vi "LS372_only_readout_Monitor.vi"() -> ()   [LabVIEW 2019]
uses:
  Utility/LS372/LS372_read_only-Cluster.ctl
  Global/Global Variables/Data_Display_global.vi
  Instrument_Setup.vi
  Equipment/Lake Shore 372/Lake Shore 372.lvlib
panel:
  in  "stop":bool
  out "LS372_only_read-Cluster":T1
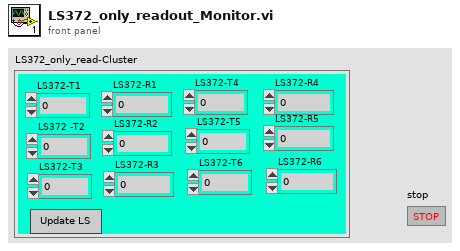
[diagram p1: front panel]
types:
  T1 = typedef "LS372_read_only-Cluster.ctl" = cluster{"LS372-T1":dbl, "LS372 -T2":dbl, "LS372-T4":dbl, "LS372-T5":dbl, "LS372-T6":dbl, "LS372-R1 ":dbl, "LS372-R2":dbl, "LS372-R3 ":dbl, "LS372-R4 \n\n\n\n":dbl, "LS372-R5":dbl, "LS372-R6 ":dbl, "LS372-T3":dbl, "Update Lakeshores":bool}
  T2 = typedef "LS372_read_only-Control.ctl" = cluster{"Update Lakeshores":bool}
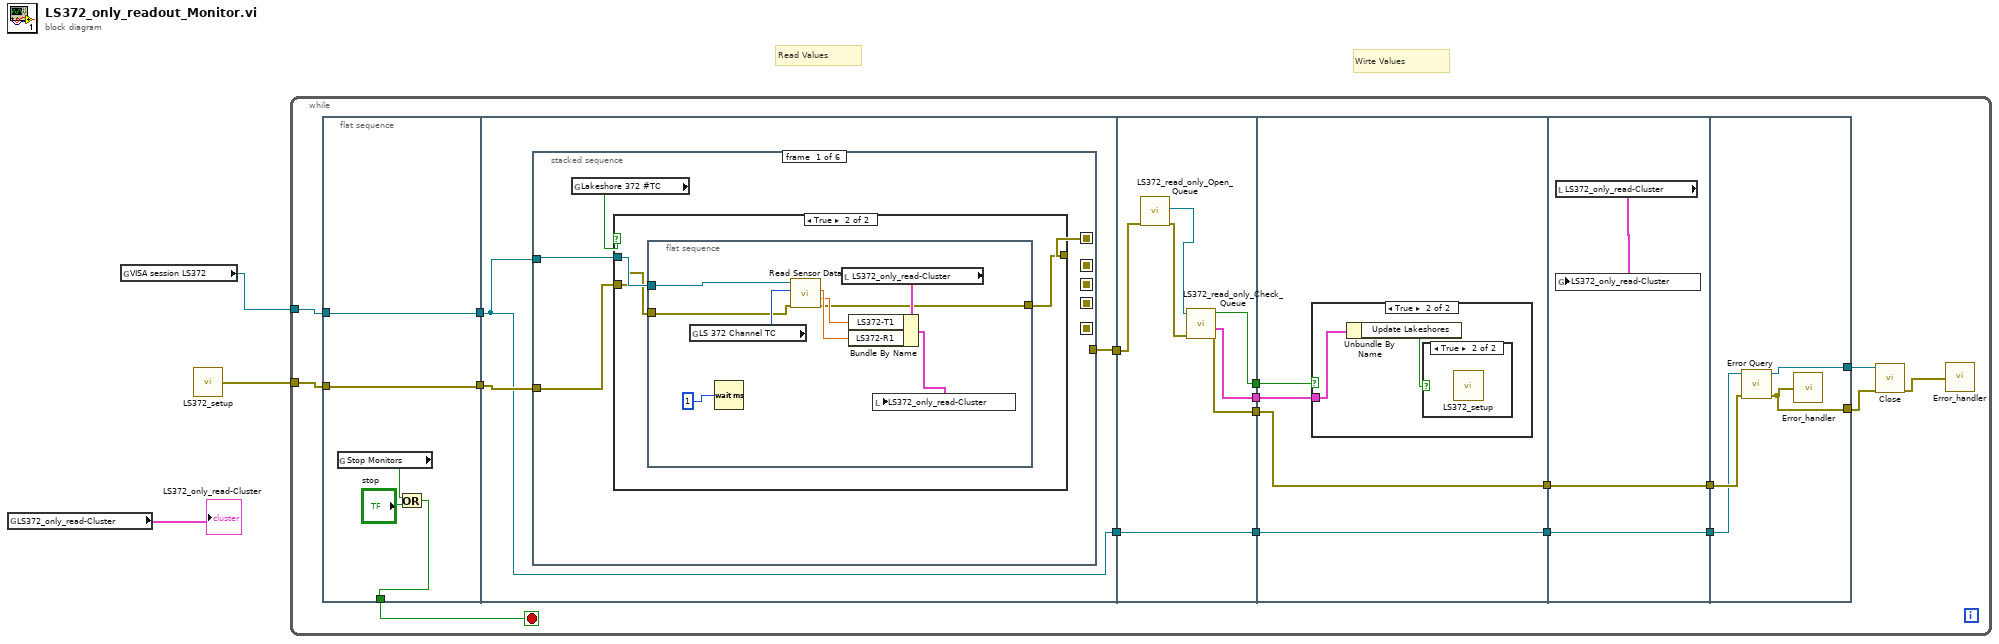
[diagram p0: block diagram]
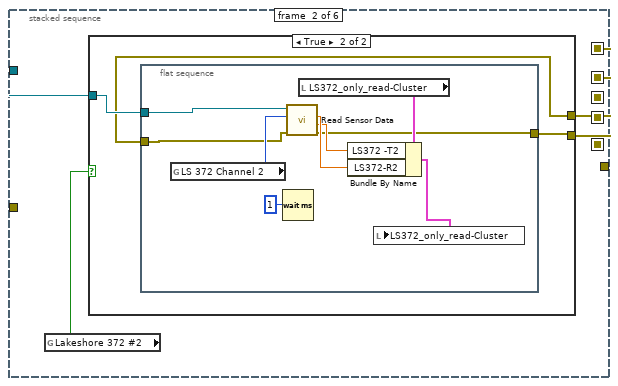
[diagram p3: hidden frame]
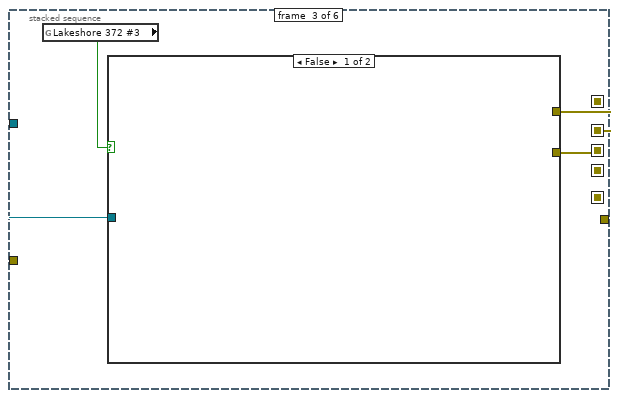
[diagram p5: hidden frame]
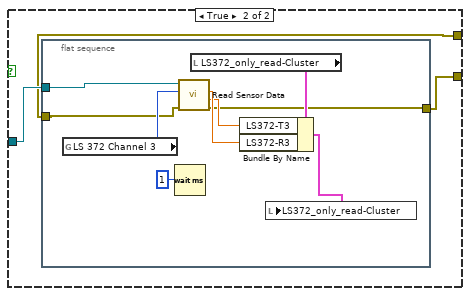
[diagram p6: hidden frame]
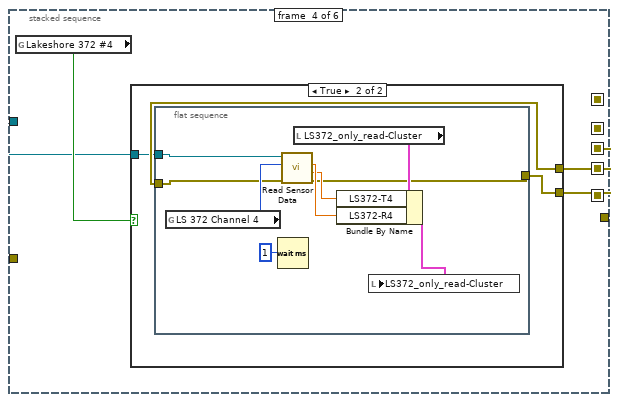
[diagram p7: hidden frame]
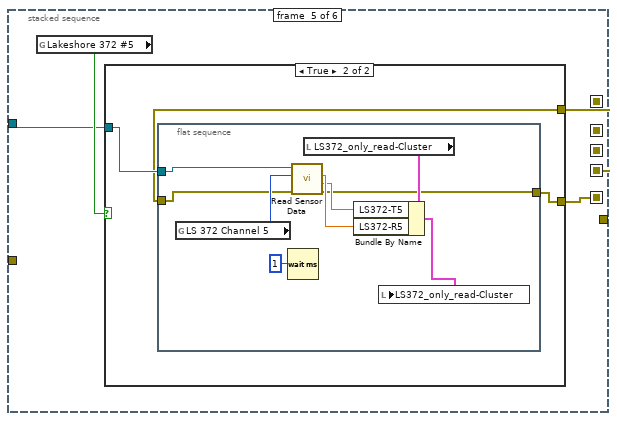
[diagram p9: hidden frame]
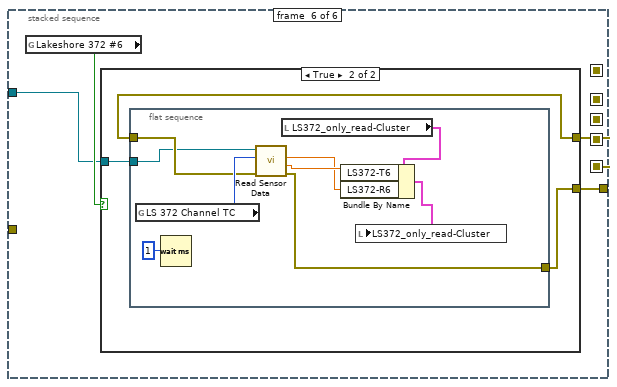
[diagram p11: hidden frame]
diagram:
  # "Wirte Values"
  # "Read Values"
  n1 = global read "Data_Display_global.vi" "LS372_only_read-Cluster"() -> (→"LS372_only_read-Cluster":T1)
  n2 = global read "Instrument_Setup.vi" "VISA session LS372"() -> (w2:refnum<visa-resource-name>)
  n3 = call "LS372_setup.vi"() -> ("error out"=w1:errorcluster)
  n4 = while {
    tunnel: w2 -> [w17]
    tunnel: w1 -> [w19]
    stop <- w21 stop-if-true
    n5 = flat-sequence {
      tunnel: [w24] -> w21
      tunnel: [w23] -> w20
      tunnel: w19 -> [w23]
      tunnel: [w22] -> w18
      tunnel: w17 -> [w22]
      tunnel: w20 -> [w29]
      tunnel: w18 -> [w27]
      tunnel: [w28] -> w16
      tunnel: [w27] -> w11
      tunnel: w16 -> [w138]
      tunnel: [w135] -> w15
      tunnel: [w134] -> w14
      tunnel: [w133] -> w13
      tunnel: w11 -> [w132]
      tunnel: [w132] -> w10
      tunnel: w15 -> [w142]
      tunnel: w14 -> [w140]
      tunnel: w13 -> [w141]
      tunnel: [w140] -> w7
      tunnel: [w139] -> w5
      tunnel: w10 -> [w139]
      tunnel: w7 -> [w147]
      tunnel: [w147] -> w6
      tunnel: w5 -> [w146]
      tunnel: [w146] -> w4
      tunnel: w6 -> [w150]
      tunnel: w4 -> [w149]
      tunnel: [w151] -> w9
      tunnel: [w148] -> w8
      frame #0 {
        n6 = global read "Data_Display_global.vi" "Stop Monitors"() -> (w26:bool)
        n7 = Or(x=w26, y="stop") -> (x .or. y?=w24:bool)
      }
      frame #1 {
        n8 = stacked-sequence {
          seq-local: [w30 _ _ _ _ _] -> [_ w50 _ _ _ _]
          seq-local: [_ w49 _ _ _ _] -> [_ _ w67 _ _ _]
          seq-local: [_ _ w66 _ _ _] -> [_ _ _ w84 _ _]
          seq-local: [_ _ _ w83 _ _] -> [_ _ _ _ w99 _]
          seq-local: [_ _ _ _ w98 _] -> [_ _ _ _ _ w118]
          tunnel: w27 -> [w32 w48 w64 w81 w100 w115]
          tunnel: w29 -> [w31 _ _ _ _ _]
          tunnel: [_ _ _ _ _ w117] -> w28
          frame #0 {
            n9 = global read "Instrument_Setup.vi" "Lakeshore 372 #TC"() -> (w33:bool)
            n10 = case shown="True" w33 {
              tunnel: w32 -> [_ w37]
              tunnel: [w34 w35] -> w30
              tunnel: w31 -> [w34 w36]
              frame False {
              }
              frame True {
                n11 = flat-sequence {
                  tunnel: [w39] -> w35
                  tunnel: w37 -> [w46]
                  tunnel: w36 -> [w42]
                  frame #0 {
                    n12 = global read "Instrument_Setup.vi" "LS 372 Channel TC"() -> (w45:u16)
                    n13 = Wait (ms)(milliseconds to wait=1) -> ()  [unwired: 1 out]
                    n14 = call "Read Sensor Data.vi"("error in (no error)"=w42, "Channel (1:1)"=w45, "VISA resource name"=w46) -> ("error out"=w39:errorcluster, "Kelvin Reading"=w43:dbl, "Resistance Reading"=w44:dbl)  [unwired: 3 in, 3 out]
                    n15 = local read "LS372_only_read-Cluster"() -> (w41:T1)
                    n16 = Bundle By Name(cluster=w41, "LS372-T1"=w43, "LS372-R1"=w44) -> (w40:T1)
                    n17 = local write "LS372_only_read-Cluster"(w40) -> ()
                  }
                }
              }
            }
          }
          frame #1 {
            n18 = global read "Instrument_Setup.vi" "Lakeshore 372 #2"() -> (w47:bool)
            n19 = case shown="True" w47 {
              tunnel: w50 -> [w51 w52]
              tunnel: [w51 w53] -> w49
              tunnel: w48 -> [_ w54]
              frame False {
              }
              frame True {
                n20 = flat-sequence {
                  tunnel: [w55] -> w53
                  tunnel: w54 -> [w62]
                  tunnel: w52 -> [w58]
                  frame #0 {
                    n21 = global read "Instrument_Setup.vi" "LS 372 Channel 2"() -> (w61:u16)
                    n22 = Wait (ms)(milliseconds to wait=1) -> ()  [unwired: 1 out]
                    n23 = call "Read Sensor Data.vi"("error in (no error)"=w58, "Channel (1:1)"=w61, "VISA resource name"=w62) -> ("error out"=w55:errorcluster, "Kelvin Reading"=w59:dbl, "Resistance Reading"=w60:dbl)  [unwired: 3 in, 3 out]
                    n24 = local read "LS372_only_read-Cluster"() -> (w57:T1)
                    n25 = Bundle By Name(cluster=w57, "LS372 -T2"=w59, "LS372-R2"=w60) -> (w56:T1)
                    n26 = local write "LS372_only_read-Cluster"(w56) -> ()
                  }
                }
              }
            }
          }
          frame #2 {
            n27 = global read "Instrument_Setup.vi" "Lakeshore 372 #3"() -> (w65:bool)
            n28 = case shown="False" w65 {
              tunnel: w67 -> [w68 w70]
              tunnel: [w68 w69] -> w66
              tunnel: w64 -> [_ w71]
              frame False {
              }
              frame True {
                n29 = flat-sequence {
                  tunnel: [w72] -> w69
                  tunnel: w70 -> [w75]
                  tunnel: w71 -> [w79]
                  frame #0 {
                    n30 = global read "Instrument_Setup.vi" "LS 372 Channel 3"() -> (w78:u16)
                    n31 = Wait (ms)(milliseconds to wait=1) -> ()  [unwired: 1 out]
                    n32 = call "Read Sensor Data.vi"("error in (no error)"=w75, "Channel (1:1)"=w78, "VISA resource name"=w79) -> ("error out"=w72:errorcluster, "Kelvin Reading"=w76:dbl, "Resistance Reading"=w77:dbl)  [unwired: 3 in, 3 out]
                    n33 = local read "LS372_only_read-Cluster"() -> (w74:T1)
                    n34 = Bundle By Name(cluster=w74, "LS372-T3"=w76, "LS372-R3"=w77) -> (w73:T1)
                    n35 = local write "LS372_only_read-Cluster"(w73) -> ()
                  }
                }
              }
            }
          }
          frame #3 {
            n36 = global read "Instrument_Setup.vi" "Lakeshore 372 #4"() -> (w82:bool)
            n37 = case shown="True" w82 {
              tunnel: w84 -> [w85 w87]
              tunnel: [w85 w88] -> w83
              tunnel: w81 -> [_ w86]
              frame False {
              }
              frame True {
                n38 = flat-sequence {
                  tunnel: [w89] -> w88
                  tunnel: w86 -> [w96]
                  tunnel: w87 -> [w92]
                  frame #0 {
                    n39 = global read "Instrument_Setup.vi" "LS 372 Channel 4"() -> (w95:u16)
                    n40 = Wait (ms)(milliseconds to wait=1) -> ()  [unwired: 1 out]
                    n41 = call "Read Sensor Data.vi"("error in (no error)"=w92, "Channel (1:1)"=w95, "VISA resource name"=w96) -> ("error out"=w89:errorcluster, "Kelvin Reading"=w93:dbl, "Resistance Reading"=w94:dbl)  [unwired: 3 in, 3 out]
                    n42 = local read "LS372_only_read-Cluster"() -> (w91:T1)
                    n43 = Bundle By Name(cluster=w91, "LS372-T4"=w93, "LS372-R4"=w94) -> (w90:T1)
                    n44 = local write "LS372_only_read-Cluster"(w90) -> ()
                  }
                }
              }
            }
          }
          frame #4 {
            n45 = global read "Instrument_Setup.vi" "Lakeshore 372 #5"() -> (w101:bool)
            n46 = case shown="True" w101 {
              tunnel: w100 -> [_ w105]
              tunnel: w99 -> [w102 w104]
              tunnel: [w102 w103] -> w98
              frame False {
              }
              frame True {
                n47 = flat-sequence {
                  tunnel: [w106] -> w103
                  tunnel: w105 -> [w113]
                  tunnel: w104 -> [w109]
                  frame #0 {
                    n48 = global read "Instrument_Setup.vi" "LS 372 Channel 5"() -> (w112:u16)
                    n49 = Wait (ms)(milliseconds to wait=1) -> ()  [unwired: 1 out]
                    n50 = call "Read Sensor Data.vi"("error in (no error)"=w109, "Channel (1:1)"=w112, "VISA resource name"=w113) -> ("error out"=w106:errorcluster, "Kelvin Reading"=w110:dbl, "Resistance Reading"=w111:dbl)  [unwired: 3 in, 3 out]
                    n51 = local read "LS372_only_read-Cluster"() -> (w108:T1)
                    n52 = Bundle By Name(cluster=w108, "LS372-T5"=w110, "LS372-R5"=w111) -> (w107:T1)
                    n53 = local write "LS372_only_read-Cluster"(w107) -> ()
                  }
                }
              }
            }
          }
          frame #5 {
            n54 = global read "Instrument_Setup.vi" "Lakeshore 372 #6"() -> (w116:bool)
            n55 = case shown="True" w116 {
              tunnel: w118 -> [w119 w121]
              tunnel: [w119 w120] -> w117
              tunnel: w115 -> [_ w122]
              frame False {
              }
              frame True {
                n56 = flat-sequence {
                  tunnel: [w123] -> w120
                  tunnel: w122 -> [w128]
                  tunnel: w121 -> [w129]
                  frame #0 {
                    n57 = global read "Instrument_Setup.vi" "LS 372 Channel TC"() -> (w130:u16)
                    n58 = Wait (ms)(milliseconds to wait=1) -> ()  [unwired: 1 out]
                    n59 = call "Read Sensor Data.vi"("error in (no error)"=w129, "Channel (1:1)"=w130, "VISA resource name"=w128) -> ("error out"=w123:errorcluster, "Kelvin Reading"=w125:dbl, "Resistance Reading"=w124:dbl)  [unwired: 3 in, 3 out]
                    n60 = local read "LS372_only_read-Cluster"() -> (w127:T1)
                    n61 = Bundle By Name(cluster=w127, "LS372-T6"=w125, "LS372-R6"=w124) -> (w126:T1)
                    n62 = local write "LS372_only_read-Cluster"(w126) -> ()
                  }
                }
              }
            }
          }
        }
      }
      frame #2 {
        n63 = call "LS372_read_only_Open_Queue.vi"("error in (no error)"=w138) -> ("error out"=w136:errorcluster, "queue out"=w137:refnum<queue>)  [unwired: 9 in]
        n64 = call "LS372_read_only_Check_Queue.vi"("error in (no error)"=w136, "queue"=w137) -> ("error out"=w134:errorcluster, "LS372_only_read-Cluster Control"=w133:T2, "New Entries?"=w135:bool)  [unwired: 6 in]
      }
      frame #3 {
        n65 = case shown="True" w142 {
          tunnel: w141 -> [_ w144]
          frame False {
          }
          frame True {
            n66 = Unbundle By Name(w144) -> ("Update Lakeshores"=w143:bool)
            n67 = case shown="True" w143 {
              frame False {
              }
              frame True {
                n68 = call "LS372_setup.vi"() -> ()  [unwired: 1 out]
              }
            }
          }
        }
      }
      frame #4 {
        n69 = local read "LS372_only_read-Cluster"() -> (w145:T1)
        n70 = global write "Data_Display_global.vi" "LS372_only_read-Cluster"(w145) -> ()
      }
      frame #5 {
        n71 = call "Error Query.vi"("error in (no error)"=w150, "VISA resource name"=w149) -> ("error out"=w148:errorcluster, "VISA resource name out"=w151:refnum<visa-resource-name>)  [unwired: 7 in, 1 out]
        n72 = call "Error_handler.vi"("error constant"=w148) -> ()
      }
    }
    n73 = call "Close.vi"("error in (no error)"=w8, "VISA resource name"=w9) -> ("error out"=w12:errorcluster)  [unwired: 9 in]
    n74 = call "Error_handler.vi"("error constant"=w12) -> ()
  }
